vi "Read From File.vi"(8 "error in (no error)":errorcluster, 11 "file path":path) -> (0 "error out":errorcluster, 2 "digital serial input settings":T1={"number of channels"=0, "data justification"=enum."Left Justified", "endianness"=enum."LSB First", "channel length"=0, "bit depth"=0, "frame clock rate"=0.0, "bit clock edge sync"=enum."Falling", "master clock source"=enum."Internal", "master clock rate"=0.0, "Logic Level"=enum."1.2 V", "frame sync edge for channel 0"=enum."Rising", "Channel 0 Offset"=0}, 5 "file exists?":bool)   [LabVIEW 2022 SP3, in "Digital Serial Input Settings.lvlib"]
uses:
  Digital Serial Input Settings.lvlib
  controls/digital serial input settings.ctl
  <vilib>/PDM Acquisition Toolkit/shared/controls/PCM Data Justification.ctl
  <vilib>/PDM Acquisition Toolkit/shared/controls/PCM Bit Endianness.ctl
  <vilib>/PDM Acquisition Toolkit/shared/controls/Digital Edge.ctl
  controls/digital audio protocol/master clock source.ctl
  <vilib>/PDM Acquisition Toolkit/host/Classes/Session/Controls/Logic Levels.ctl
  digital serial input settings_json.ctl
  <vilib>/PDM Acquisition Toolkit/shared/PDM Shared.lvlib
  <vilib>/PDM Acquisition Toolkit/host/Classes/Session/DecoderSession.lvclass
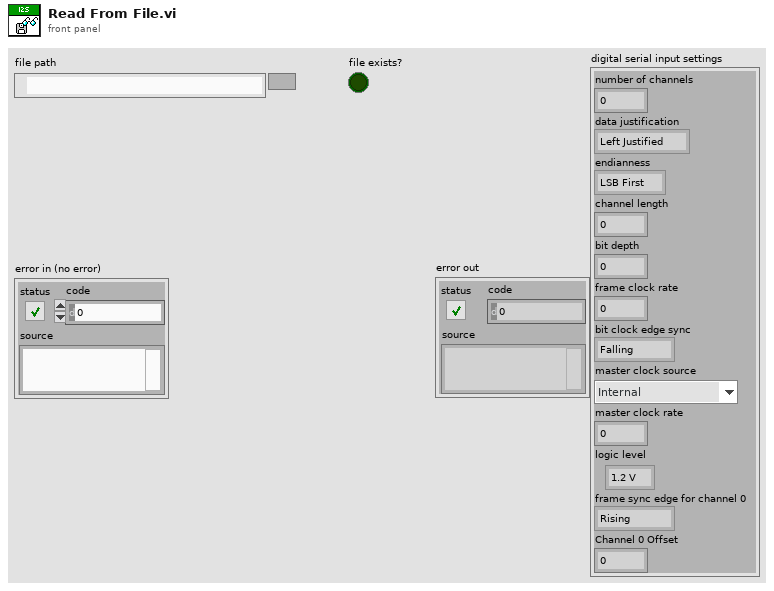
[diagram p1: front panel]
types:
  T1 = typedef "digital serial input settings.ctl" = cluster{"number of channels":u32, "data justification":T2, "endianness":T3, "channel length":u32, "bit depth":u32, "frame clock rate":dbl, "bit clock edge sync":T4, "master clock source":T5, "master clock rate":dbl, "Logic Level":T6, "frame sync edge for channel 0":T4, "Channel 0 Offset":u32}
  T2 = typedef "PDM Shared.lvlib/PCM Data Justification.ctl" = enum16{"Left Justified", "Right Justified"}
  T3 = typedef "PDM Shared.lvlib/PCM Bit Endianness.ctl" = enum16{"MSB First", "LSB First"}
  T4 = typedef "PDM Shared.lvlib/Digital Edge.ctl" = enum8{"Rising", "Falling"}
  T5 = typedef "master clock source.ctl" = enum32{"Internal", "External"}
  T6 = typedef "PDM Acquisition Class Library.lvlib/DecoderSession.lvclass/Logic Levels.ctl" = enum16{"3.3 V", "1.8 V", "1.2 V"}
  T7 = typedef "Digital Serial Input Settings.lvlib/digital serial input settings_json.ctl" = cluster{"number of channels":u32, "data justification":string, "endianness":string, "channel length":u32, "bit depth":u32, "frame clock rate":dbl, "bit clock edge sync":string, "master clock souce":string, "master clock rate":dbl, "logic level":string, "frame sync edge for channel 0":string, "Channel 0 Offset":u32}
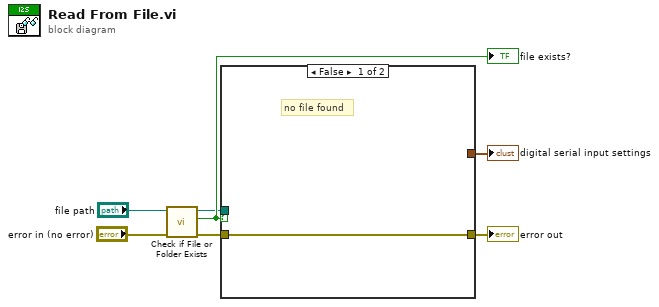
[diagram p0: block diagram]
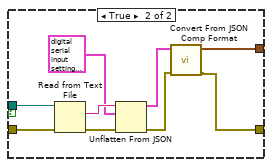
[diagram p2: hidden frame]
diagram:
  n1 = call <vilib>:"Check if File or Folder Exists.vi"("error in (no error)"="error in (no error)", "path"="file path") -> ("error out"=w6:errorcluster, "file or folder exists?"=w5:bool, "dup path"=w4:path)  [unwired: 7 in]
  "file exists?" <- w5
  n2 = case shown="False" w5 {
    tunnel: w6 -> [w8 w16]
    tunnel: w4 -> [_ w17]
    tunnel: [_ w9] -> w1
    tunnel: [w8 w12] -> w2
    frame False {
      # "no file found"
    }
    frame True {
      n3 = Read from Text File(file (use dialog)=w17, error in=w16) -> (text=w14:string, error out=w15:errorcluster)  [unwired: 2 in, 2 out]
      n4 = Unflatten From JSON(JSON string=w14, type and defaults=T7 {"number of channels"=51200, "data justification"="", "endianness"="", "channel length"=5, "bit depth"=0, "frame clock rate"=0.0, "bit clock edge sync"="", "master clock souce"="", "master clock rate"=0.0, "logic level"="", "frame sync edge for channel 0"="", "Channel 0 Offset"=0} ("output settings"), error in (no error)=w15) -> (value=w10:T7, error out=w13:errorcluster)  [unwired: 4 in]
      n5 = call "Convert From JSON Comp Format.vi"("error in (no error)"=w13, "input settings JSON"=w10) -> ("error out"=w12:errorcluster, "input settings"=w9:T1)  [unwired: 8 in]
    }
  }
  "error out" <- w2
  "digital serial input settings" <- w1
